vi "generate image arrays.vi"() -> (3 "Image Arrays":T1)   [LabVIEW 2017]
uses:
  controls/image arrays.ctl
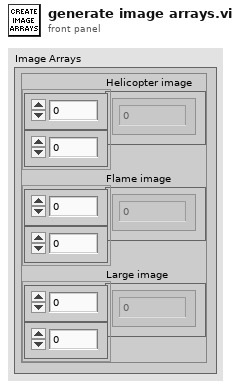
[diagram p1: front panel]
types:
  T1 = typedef "image arrays.ctl" = cluster{"Helicopter image":u8[][], "Flame image":u8[][], "Large image":u8[][]}
  T2 = typedef "Image Type" = u32
  T3 = typedef "IMAQ Image.ctl" = refnum<image>
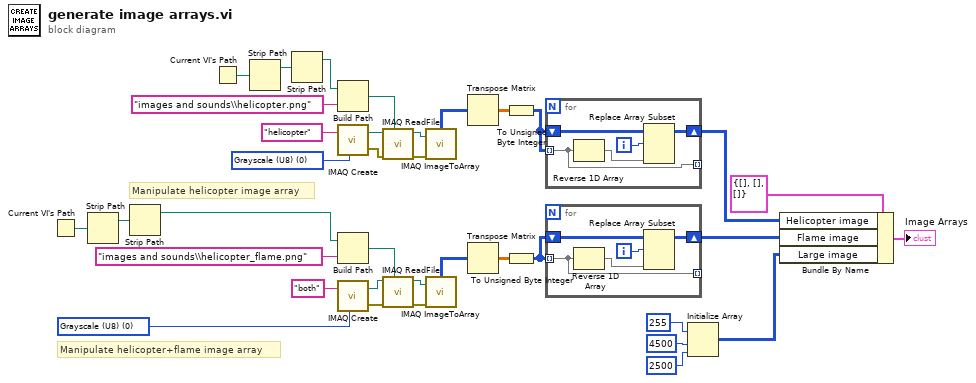
[diagram p0: block diagram]
diagram:
  w30 = T2 0 items=["Grayscale (U8)", "Grayscale (I16)", "Grayscale (SGL)", "Complex (CSG)", "RGB (U32)", "HSL (U32)", "RGB (U64)", "Grayscale (U16)"] ("Image Type")
  w17 = T2 0 items=["Grayscale (U8)", "Grayscale (I16)", "Grayscale (SGL)", "Complex (CSG)", "RGB (U32)", "HSL (U32)", "RGB (U64)", "Grayscale (U16)"] ("Image Type")
  # "Manipulate helicopter+flame image array"
  # "Manipulate helicopter image array"
  n1 = Current VI's Path() -> (path=w27:path)
  n2 = Strip Path(path=w27) -> (stripped path=w26:path)  [unwired: 1 out]
  n3 = Strip Path(path=w26) -> (stripped path=w1:path)  [unwired: 1 out]
  n4 = Current VI's Path() -> (path=w20:path)
  n5 = Strip Path(path=w20) -> (stripped path=w21:path)  [unwired: 1 out]
  n6 = Strip Path(path=w21) -> (stripped path=w2:path)  [unwired: 1 out]
  n7 = Build Path(base path=w2, name or relative path="images and sounds\\helicopter.png") -> (appended path=w23:path)
  n8 = call "IMAQ Create"("Image Name"="helicopter", "Image Type"=w17) -> ("New Image"=w12:T3, "error out"=w14:errorcluster)  [unwired: 3 in]
  n9 = Build Path(base path=w1, name or relative path="images and sounds\\helicopter_flame.png") -> (appended path=w24:path)
  n10 = call "IMAQ Create"("Image Name"="both", "Image Type"=w30) -> ("New Image"=w35:T3, "error out"=w33:errorcluster)  [unwired: 3 in]
  n11 = call "IMAQ ReadFile"("File Path"=w23, "error in (no error)"=w14, "Image"=w12) -> ("error out"=w15:errorcluster, "Image Out"=w16:T3)  [unwired: 4 in, 3 out]
  n12 = call "IMAQ ReadFile"("File Path"=w24, "error in (no error)"=w33, "Image"=w35) -> ("error out"=w32:errorcluster, "Image Out"=w31:T3)  [unwired: 4 in, 3 out]
  n13 = call "IMAQ ImageToArray"("error in (no error)"=w15, "Image"=w16) -> ("Image Pixels (U8)"=w11:u8[][])  [unwired: 2 in, 4 out]
  n14 = call "IMAQ ImageToArray"("error in (no error)"=w32, "Image"=w31) -> ("Image Pixels (U8)"=w36:u8[][])  [unwired: 2 in, 4 out]
  n15 = Transpose Matrix(1:w11) -> (0:w18:dbl[][])
  n16 = Transpose Matrix(1:w36) -> (0:w29:dbl[][])
  n17 = To Unsigned Byte Integer(number=w18) -> (unsigned 8bit integer=w19:u8[][])
  n18 = To Unsigned Byte Integer(number=w29) -> (unsigned 8bit integer=w28:u8[][])
  n19 = for {
    tunnel: [w41] -> _ mode=indexing
    tunnel: w19 -> [w41] mode=indexing
    shift-right: [w39] -> w8
    shift-left: w19 -> [w40]
    i -> [w37]
    n20 = Reverse 1D Array(array=w41) -> (reversed array=w38:u8[])
    n21 = Replace Array Subset(array=w40, new element=w38, index (row)=w37) -> (w39:u8[][])  [unwired: 1 in]
  }
  n22 = for {
    tunnel: [w46] -> _ mode=indexing
    tunnel: w28 -> [w46] mode=indexing
    shift-right: [w44] -> w7
    shift-left: w28 -> [w45]
    i -> [w42]
    n23 = Reverse 1D Array(array=w46) -> (reversed array=w43:u8[])
    n24 = Replace Array Subset(array=w45, new element=w43, index (row)=w42) -> (w44:u8[][])  [unwired: 1 in]
  }
  n25 = Initialize Array(u8 255 ("element"), 4500 ("dimension size"), 2500 ("dimension size")) -> (w3:u8[][])
  n26 = Bundle By Name(cluster=T1 {"Helicopter image"=[], "Flame image"=[], "Large image"=[]} ("Image Arrays"), "Helicopter image"=w8, "Flame image"=w7, "Large image"=w3) -> (→"Image Arrays":T1)
